vi "Init SelectionList.vi"(6 "Selection Mode":T1, 7 "ListSelection in":refnum<class "ListSelection.lvclass">, 8 "error in":errorcluster, 9 "Timeout (-1)":i32=-1, 10 "Items List":string[](array[string]), 11 "Message":string) -> (0 "error out":errorcluster, 3 "ListSelection out":refnum<class "ListSelection.lvclass">)   [LabVIEW 2012, in "ListSelection.lvlib" / "ListSelection.lvclass"]
doc: "Instantiates an object of class \"Error Message Box\"."
uses:
  ListSelection.lvclass
  Selection Mode.ctl
  ListSelection.lvclass/ListSelection.ctl
  MessageBox/MessageBox.lvclass
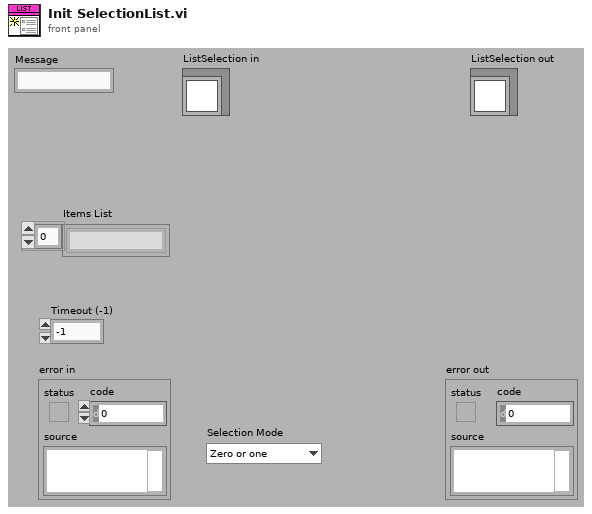
[diagram p1: front panel]
types:
  T1 = typedef "ListSelection.lvlib/ListSelection.lvclass/Selection Mode.ctl" = enum16{"Zero or one", "One", "Zero or more", "One or more"}
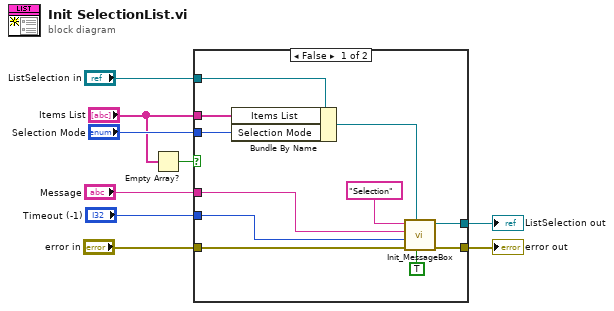
[diagram p0: block diagram]
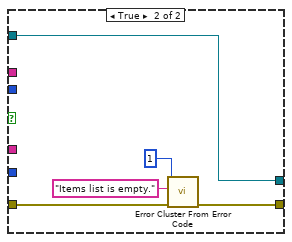
[diagram p2: hidden frame]
diagram:
  n1 = Empty Array?(array="Items List") -> (empty?=w1:bool)
  n2 = case shown="False" w1 {
    tunnel: "ListSelection in" -> [w20 w25]
    tunnel: [w18 w25] -> w8
    tunnel: "Timeout (-1)" -> [w17 _]
    tunnel: "error in" -> [w16 w24]
    tunnel: [w15 w23] -> w5
    tunnel: "Message" -> [w13 _]
    tunnel: "Selection Mode" -> [w12 _]
    tunnel: "Items List" -> [w10 _]
    frame False {
      n3 = Bundle By Name(cluster=w20, "Items List"=w10, "Selection Mode"=w12) -> (w19:refnum<class "ListSelection.lvclass">)
      n4 = call "Init_MessageBox.vi"("Allow to close? (T)"=TRUE, "MessageBox in"=w19, "error in (no error)"=w16, "Timeout (-1)"=w17, "Message"=w13, "MsgBox Title"="Selection") -> ("error out"=w15:errorcluster, "MessageBox out"=w18:refnum<class "ListSelection.lvclass">)  [unwired: 1 in, 3 out]
    }
    frame True {
      n5 = call <vilib>:"Error Cluster From Error Code.vi"("error in (no error)"=w24, "error message (\"\")"="Items list is empty." ("error message (\"\")"), "error code (0)"=1) -> ("error out"=w23:errorcluster)  [unwired: 6 in]
    }
  }
  "ListSelection out" <- w8
  "error out" <- w5
